vi "PID control - Circle working.vi"() -> ()   [LabVIEW 2017]
uses:
  <vilib>/Simulation/Scripting/Companion Diagram/SimConfigNode/SimParams.ctl
  <vilib>/Simulation/Scripting/Companion Diagram/SimConfigNode/_simSolvers.ctl
  <vilib>/Simulation/Implementation/Shared/SIMSCR Execution Mode.ctl
  <vilib>/Simulation/Param Hierarchy/Typedefs/SIMPH Param Control Actions.ctl
  <vilib>/Simulation/Implementation/Shared/NILVSim_ParamChanged.vi
  <vilib>/Simulation/Implementation/Shared/NILVSIM_BeginStep.vi
  <vilib>/Simulation/Implementation/Shared/NILVSim_Manager.vi
  <vilib>/Utility/error.llb/Clear Errors.vi
  <vilib>/Simulation/Implementation/Shared/NILVSim_FinalizeModel.vi
  <vilib>/DAQmx/read.llb/DAQmx Read (Counter DBL 1Chan 1Samp).vi
  <vilib>/DAQmx/read.llb/DAQmx Read (Digital Bool 1Line 1Point).vi
  917b7e52-755f-4d44-bea8-9e7c9beac24e.vi
  a58f9967-76f1-4ebc-ad3d-26e75a3ca160.vi
  <vilib>/DAQmx/write.llb/DAQmx Write (Analog DBL 1Chan 1Samp).vi
  <vilib>/DAQmx/create/channels.llb/DAQmx Create Channel (AO-Voltage-Basic).vi
  <vilib>/DAQmx/create/channels.llb/DAQmx Create Channel (DI-Digital Input).vi
  <vilib>/DAQmx/create/channels.llb/DAQmx Create Channel (CI-Count Edges).vi
  <vilib>/Simulation/Implementation/Shared/SIM Unbundle Sim Info.vi
  <vilib>/Simulation/Implementation/Shared/NILVSim_Initialize.vi
  <vilib>/Simulation/Utility/Implementation/NILVSim Get Time and IsAcceptedStep.vi
  <vilib>/Simulation/Implementation/Shared/SIMSH Read Queue.vi
  <vilib>/Simulation/Implementation/Shared/NILVSim_GetModelError.vi
  <vilib>/Simulation/Implementation/Shared/SIM Bundle Sim Info.vi
  <vilib>/DAQmx/miscellaneous.llb/DAQmx Fill In Error Info.vi
  <vilib>/Simulation/Implementation/XNodeFramework/SimXNode/SimX.xnode
  <vilib>/Simulation/Model Libraries/PID/SIM PID (Parallel).vi
  <vilib>/Simulation/Model Libraries/PID/SIM PID.vi
  <vilib>/Simulation/Scripting/Companion Diagram/SimConfigNode/SimDog.xnode
  <vilib>/Simulation/Model Libraries/PID/SIM PID (Academic).vi
  <vilib>/Simulation/Implementation/Shared/NI_SIM_Implementation.lvlib
panel:
  out "Boolean":bool
  in  "origin":bool
  out "Previous Y":dbl
  out "Previous X":dbl
  out "Current Y":dbl
  out "Current X":dbl
  out "previous index":dbl
  out "both/reset enter":bool
  out "reset complete":bool
  out "x circle":bool
  out "y circle":bool
  out "Point circle is drawing":dbl=1.0
  out "false":bool
  in  "Radius 2":dbl
  out "No of Points":dbl
  out "Numeric y 2":dbl
  out "Y array":dbl[](array[numeric])
  out "array Y length 2":dbl
  out "Numeric x 2":dbl
  out "X array":dbl[](array[numeric])
  out "array x Length 2":dbl
  in  "stage circle":T1(ring)
  in  "check instruc":bool
  out "x entered":dbl
  out "y enetred":dbl
  out "greater -1 x":bool
  out "less 1 x":bool
  out "direction selected":dbl
  out "at 2f":bool
  out "Step 2J":bool
  out "Step 2H":bool
  out "Shape drawing steps":enum16{"corner", "1st switch", "reverse"}(ring)
  out "Step 2D":bool
  out "Step 2C":bool
  out "c":bool
  in  "height":dbl
  in  "length":dbl
  in  "part":T2(ring)=enum."a"
  out "Step 2A":bool
  out "Step 2B":bool
  in  "Has encoders been reset?":enum16{"don't reset", "reset"}(ring)
  out "x distance currently being travelled":dbl
  out "y distance currently being travelled":dbl
  out "error calced":dbl
  out "p1 dis 2":dbl
  out "p1 dis":dbl
  out "error y":dbl
  out "calc distance y":dbl
  out "calc distanc x":dbl
  out "error x":dbl
  out "reached y":bool
  out "reached x":bool
  out "Numeric":dbl
  in  "Draw rectangle":bool
  in  "Draw circle":bool
  out "In drawing mode":bool
  in  "Right-Down":bool
  in  "Left-Up":bool
  in  "Left-Down":bool
  in  "Right-Up":bool
  in  "right":bool
  in  "left":bool
  in  "motor 2":dbl(slide)=1.5 scale=-10.0..10.0
  in  "down":bool
  in  "up":bool
  in  "Y Length":dbl=30.0
  in  "X Length":dbl=30.0
  in  "Motor 2 encoder":tag="Dev1/ctr1"
  out "Pulses M2":dbl format="%.2f"
  in  "Motor 1 encoder":tag="Dev1/ctr0"
  out "Pulses M1":dbl format="%.2f"
  out "Right":bool
  out "Bottom":bool
  out "Left":bool
  out "Top":bool
  in  "Switch 4/Line 3":tag="Dev1/port0/line3"
  in  "Switch 3/Line 2":tag="Dev1/port0/line2"
  in  "Switch 2/Line 1":tag="Dev1/port0/line1"
  in  "Switch 1/Line 0":tag="Dev1/port0/line0"
  in  "Motor stop":bool
  in  "Motor 1":tag="Dev1/ao0"
  in  "max Voltage":dbl=10.0
  in  "Min Voltage":dbl=-10.0
  in  "Motor 2":tag="Dev1/ao1"
  in  "motor 1":dbl(slide)=1.5 scale=-10.0..10.0
  in  "stop":bool
  # "-1"
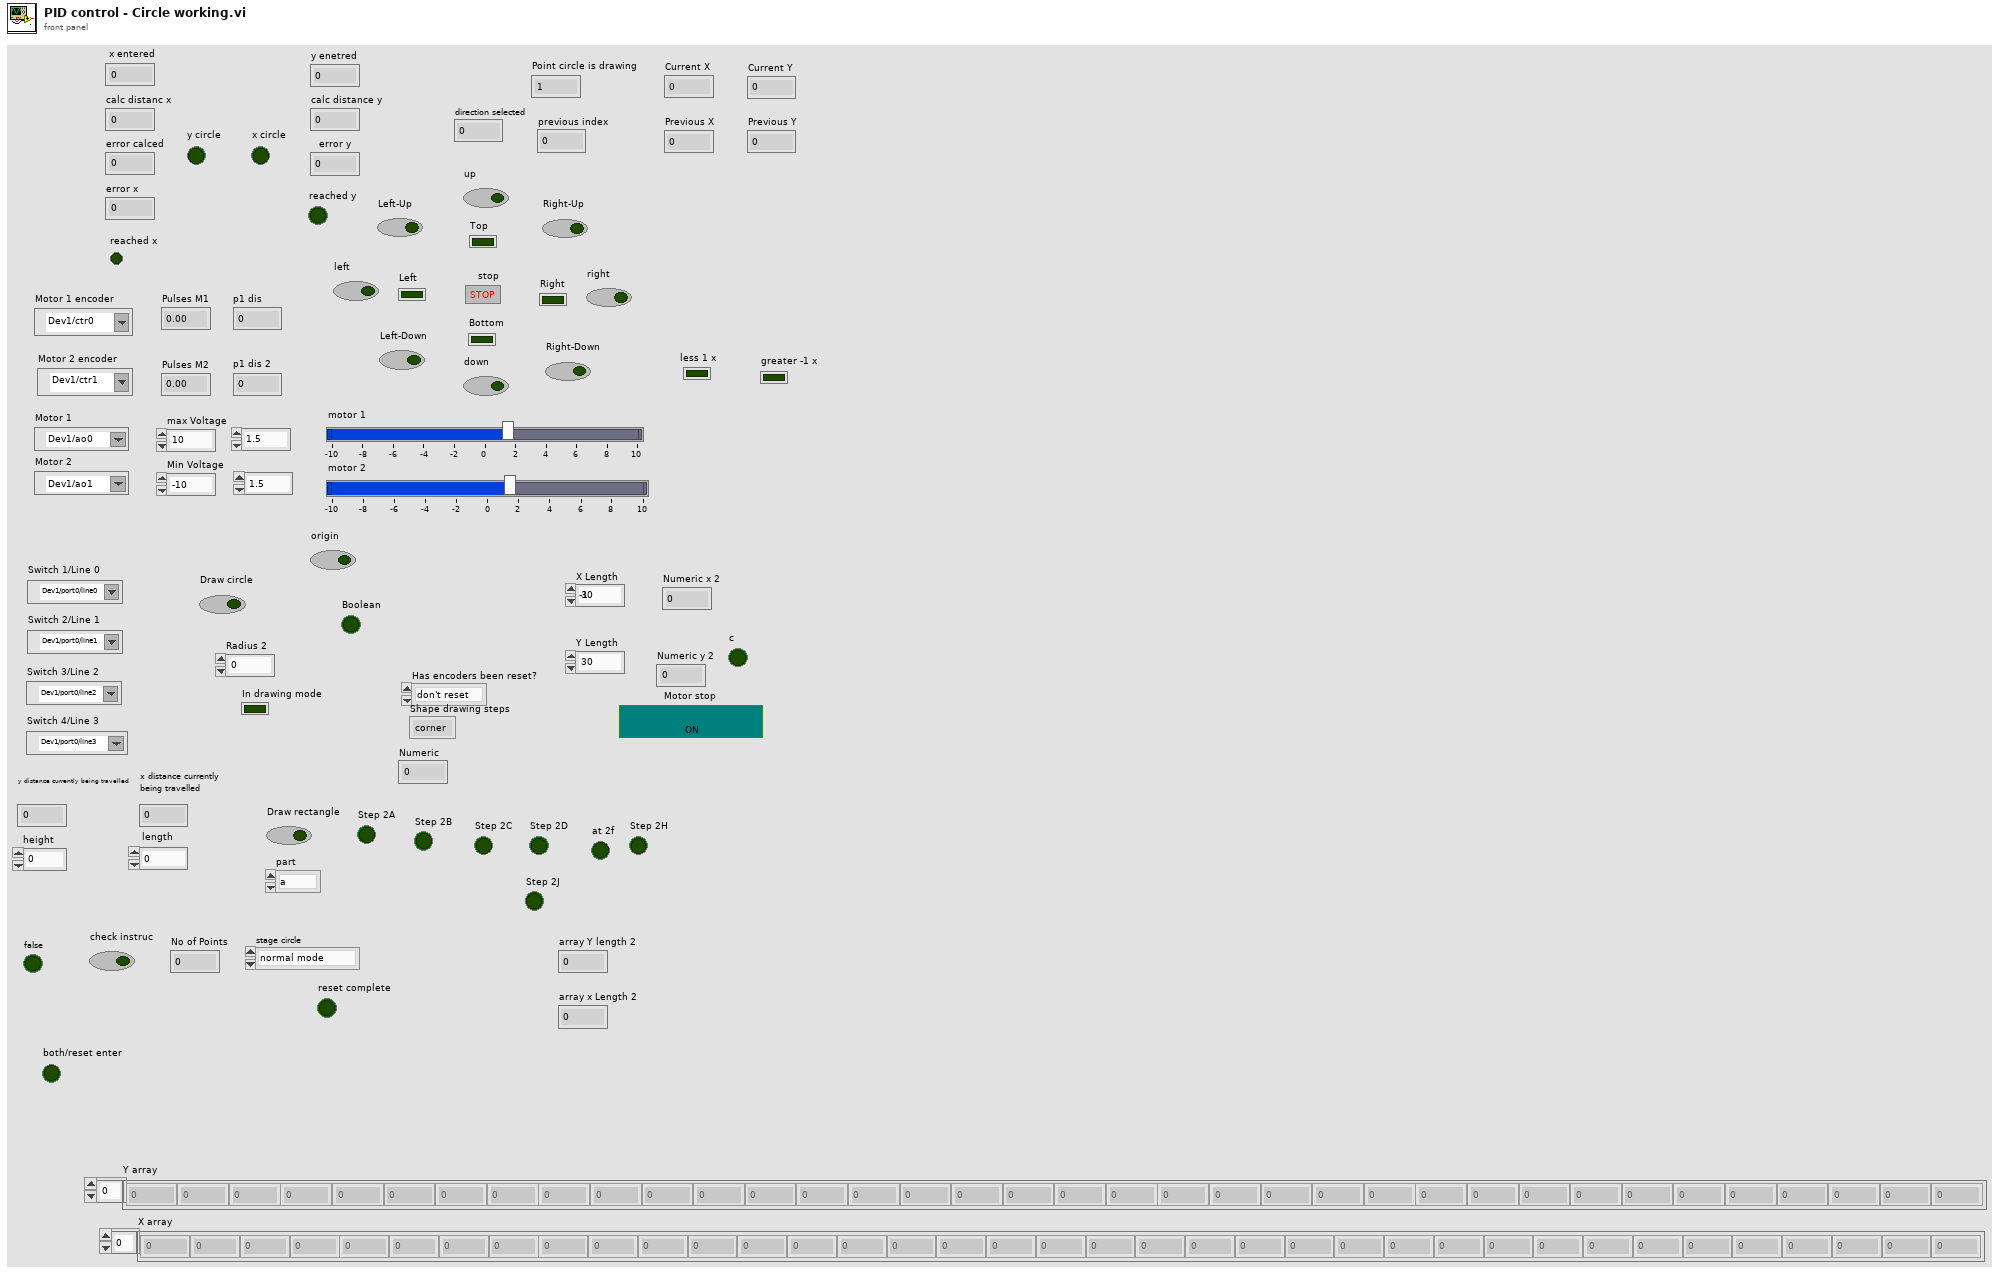
[diagram p1: front panel]
types:
  T1 = enum16{"normal mode", "create points", "draw points", "checking if draw", "reset draw counter"}
  T2 = enum16{"nothing", "j", "i", "h", "g", "f", "e", "d", "c", "b", "a"}
  T3 = enum16{"Simulate to Completion", "Single Time-Step Simulation (Fixed Step Only)"}
  T4 = typedef "SIMSCR Execution Mode.ctl" = enum16{"Simulate to Completion", "Single Time-Step Simulation (Fixed Step Only)"}
  T5 = typedef "SIMPH Param Control Actions.ctl" = enum16{"get params", "set params"}
  T6 = cluster{"SIMSH Sim Time":dbl, "SIM PID Derivative Gain.vi":cluster{"output":dbl}, "SIM PID Derivative Gain.vi - SIMSH":cluster{"SIMSH Sim Time":dbl, "t 3":dbl, "Select 2":cluster{"s? t:f":dbl}, "Equal?":cluster{"x = y?":bool}, "Or":cluster{"x .or. y?":bool}, "Equal To 0?":cluster{"x = 0?":bool}}, "High Frequency [s] (Tf)":dbl, "Gain":cluster{"output":dbl}, "Summation":cluster{"Result":dbl}, "Integral Gain - series.vi":cluster{"output":dbl}, "Integral Gain - series.vi - SIMSH":cluster{"SIMSH Sim Time":dbl, "Select 2":cluster{"s? t:f":dbl}, "integral in gain?":bool, "Integrator":cluster{"output y(t)":dbl}, "Gain 2":cluster{"output":dbl}, "Select":cluster{"s? t:f":dbl}, "Equal To 0?":cluster{"x = 0?":bool}, "Reciprocal":cluster{"1/x":dbl}}}
  T7 = typedef "SimParams.ctl" = cluster{"Initial Time (s)":dbl, "Final Time (s)":dbl, "Step Size (s)":dbl, "ODE Solver":T8, "Minimum Step Size (s)":dbl, "Maximum Step Size (s)":dbl, "Relative Tolerance":dbl, "Absolute Tolerance":dbl, "Software Timing":bool, "Initial Step Size (s)":dbl, "Automatic Fixed Step Size?":bool, "Automatic Discrete Step Size?":bool, "Discrete Step Size (s)":dbl, "Calculate using Time Step":bool, "Solver Wired?":bool, "Prev.Frm.Expected End":u64, "Prev.Frm.Actual End":u64, "Prev.Frm.Finished Late?":bool, "Prev.Iter.Expected End":u64, "Prev.Iter.Actual End":u64, "Prev.Iter.Finished Late?":bool, "Expected Iteration Start":u64, "Actual Iteration Start":u64, "Expected Frame Start":u64, "Actual Frame Start":u64, "Source Name":string, "Name":string, "Period":i64, "Deadline":i64, "Offset":i64, "Start":i64, "Priority":i32, "Timeout":i32, "Processor":i32, "Mode":enum32{"No Change", "Process missed periods, maintain original phase", "Discard missed periods, maintain original phase", "Process missed periods, ignore original phase", "Discard missed periods, ignore original phase"}, "Wakeup reason":enum32{"Normal", "Aborted", "Asynchronous wakeup", "Timing source error", "Timed loop error", "Timeout"}, "Error":errorcluster, "Source Type":string, "Secondary Source Type":string, "Global End Time":u64, "Global Start Time":u64, "Full Solver Reset":bool, "Execution Mode":T4, "Nan/Inf Check":bool, "Custom Solver Library":string, "Solver Is Variable":bool, "custom solver name":string, "Signal Collection Decimation":u32}
  T8 = typedef "_simSolvers.ctl" = enum16{"Runge-Kutta 1 (Euler)", "Runge-Kutta 2", "Runge-Kutta 3", "Runge-Kutta 4", "Runge-Kutta 23 (variable)", "Runge-Kutta 45 (variable)", "BDF (variable)", "Adams-Moulton (variable)", "Rosenbrock (variable)", "Discrete States Only", "SDIRK 4 (variable)", "Radau 5 (variable)", "Radau 9 (variable)", "Radau 13 (variable)", "Radau [Variable Order] (variable)", "Gear's Method (variable)", "Linearizer", "State Query", "Trim Eval", "Custom Solver"}
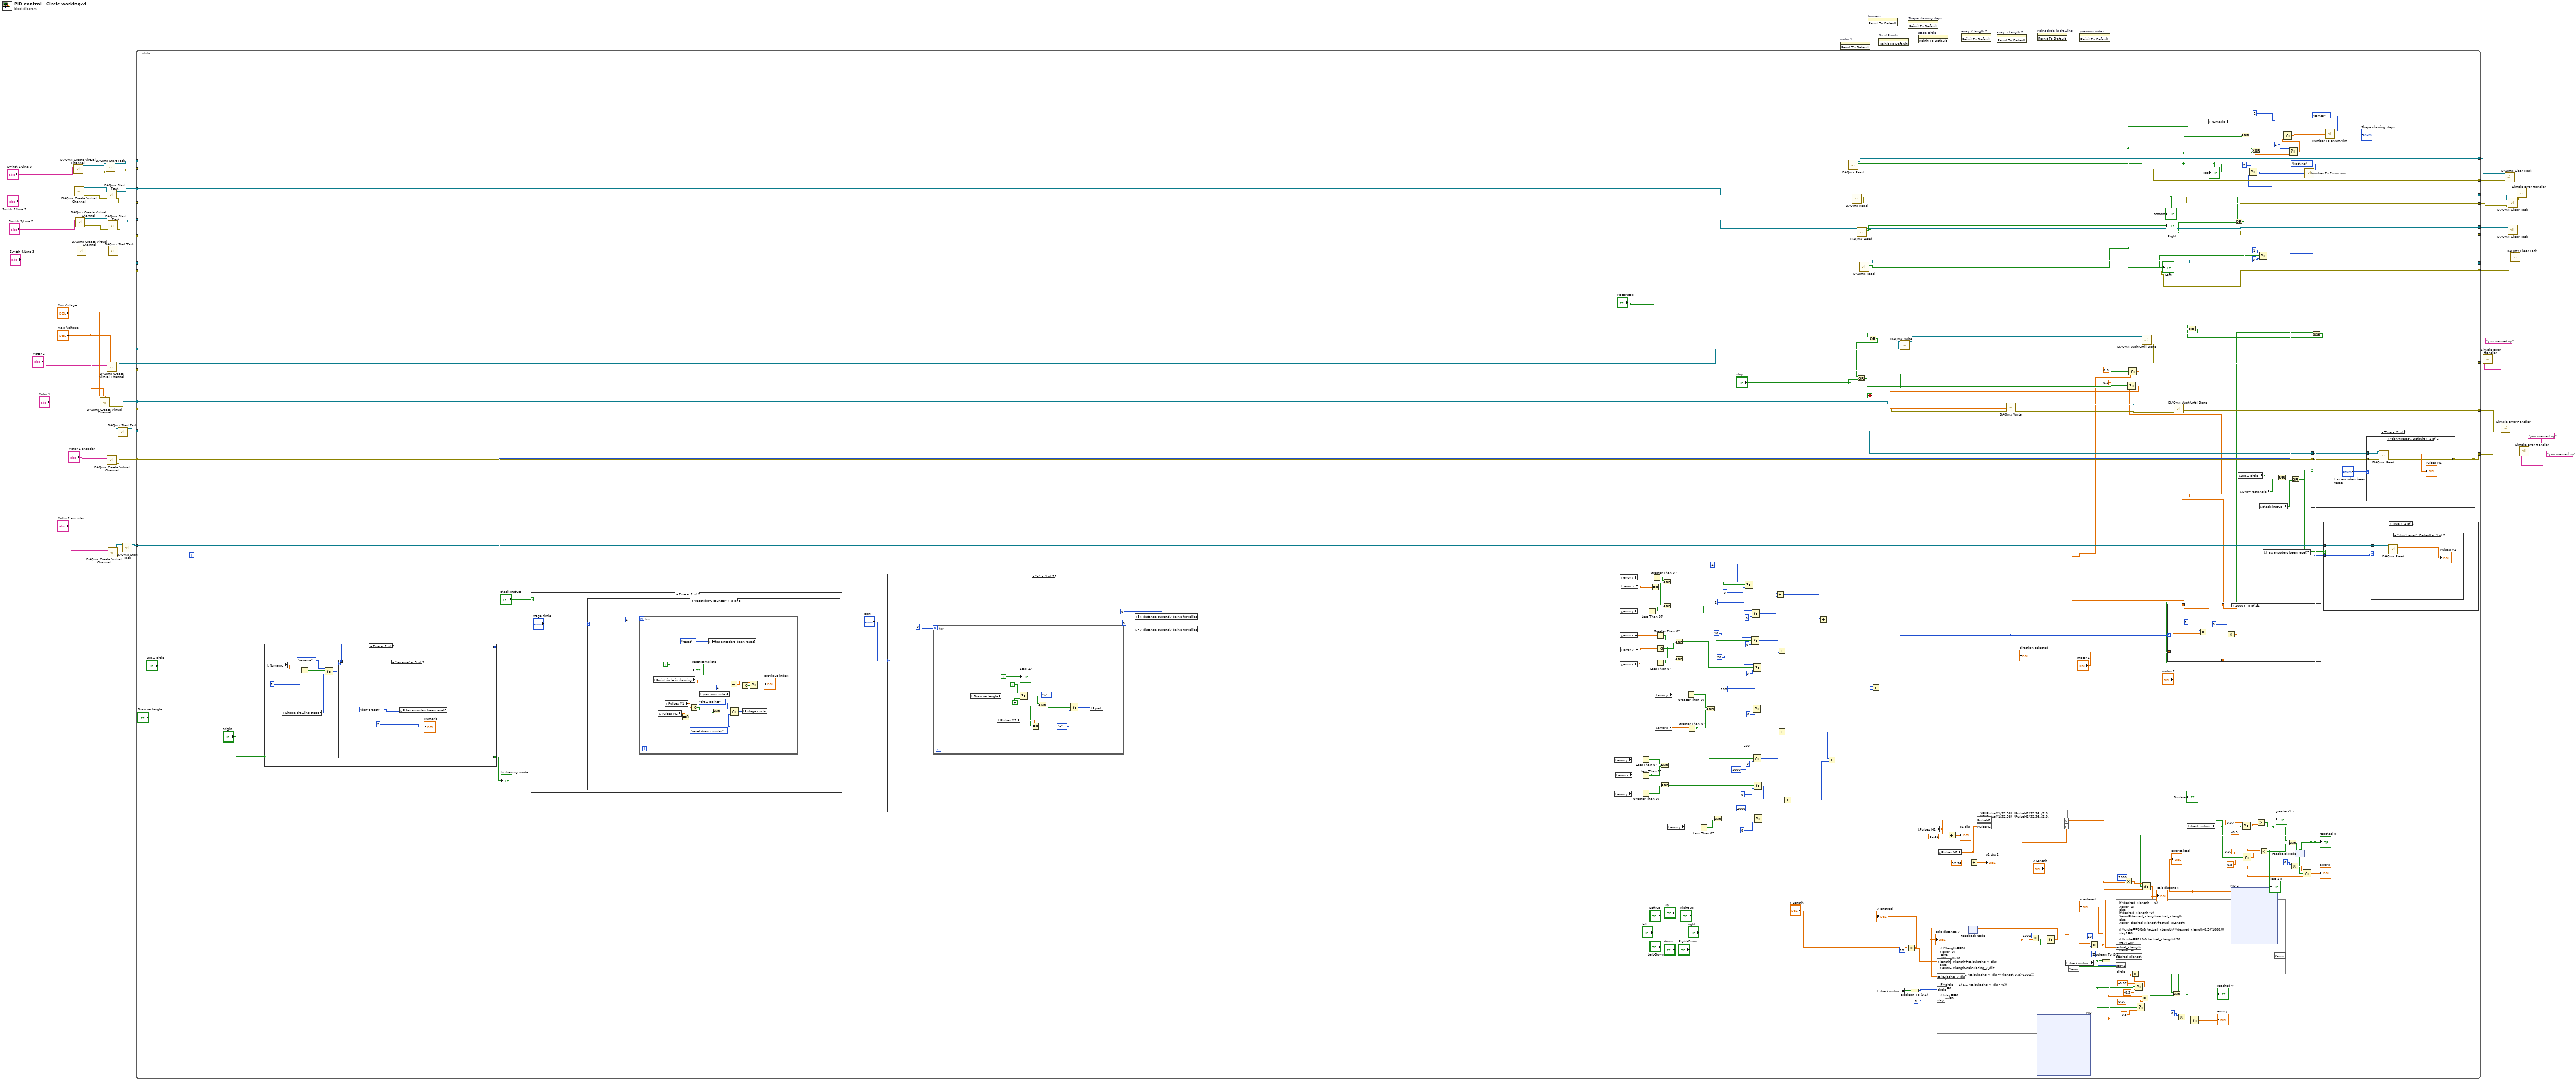
[diagram p0: block diagram]
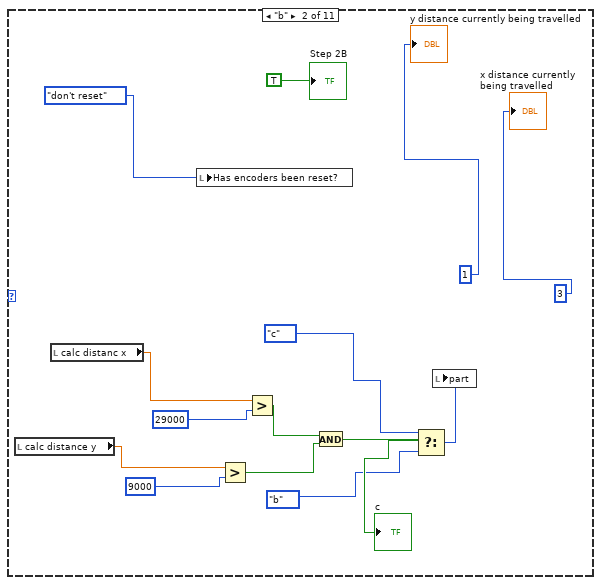
[diagram p2: hidden frame]
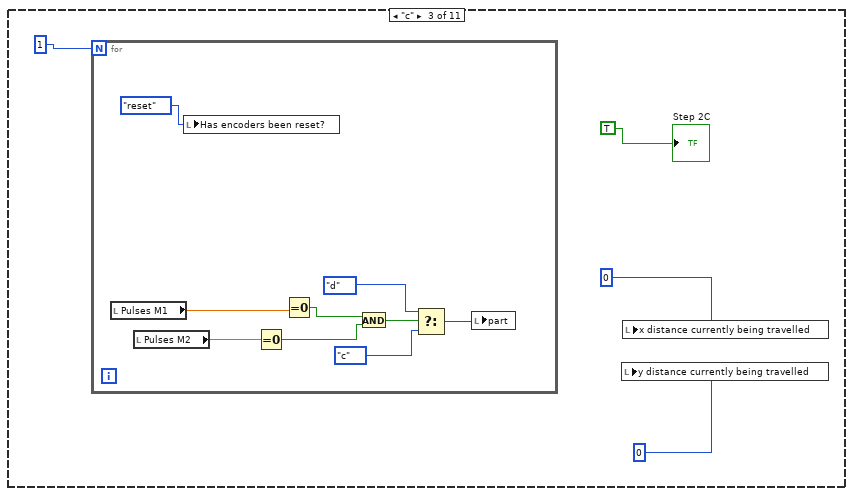
[diagram p3: hidden frame]
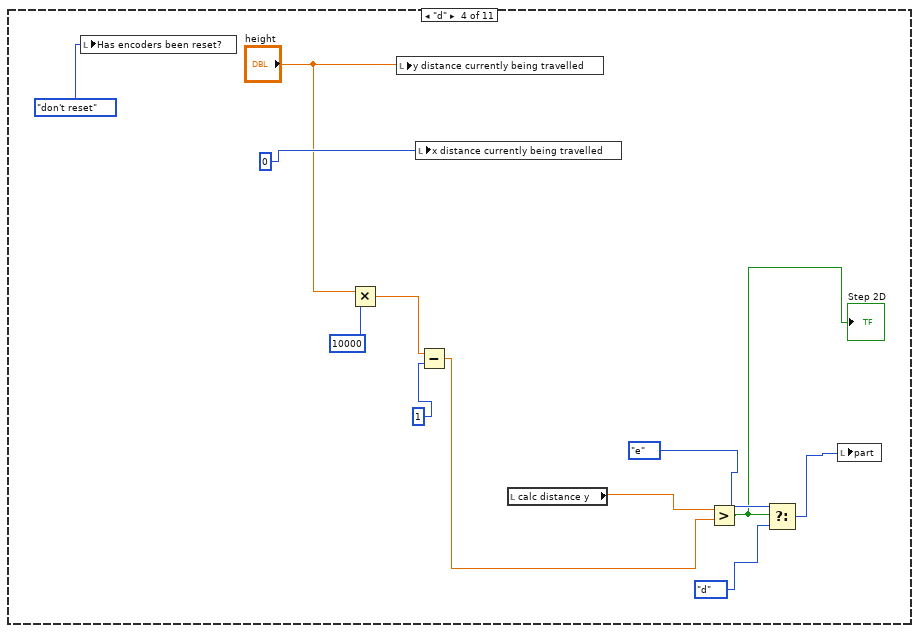
[diagram p4: hidden frame]
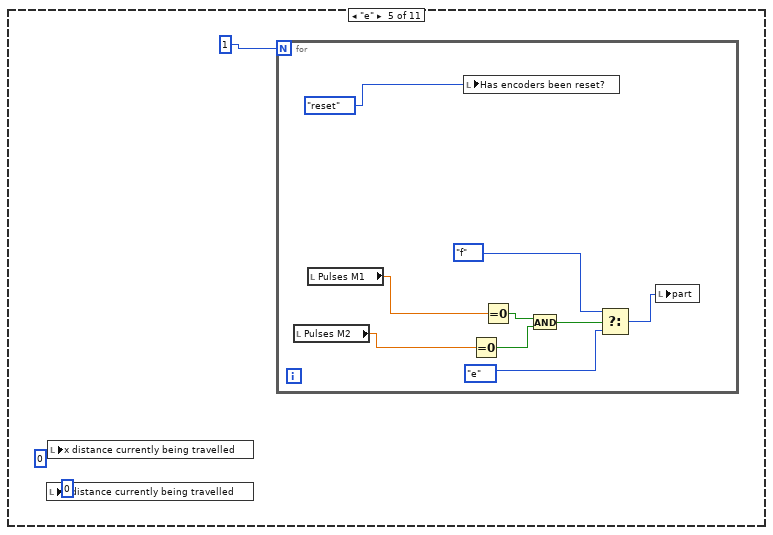
[diagram p5: hidden frame]
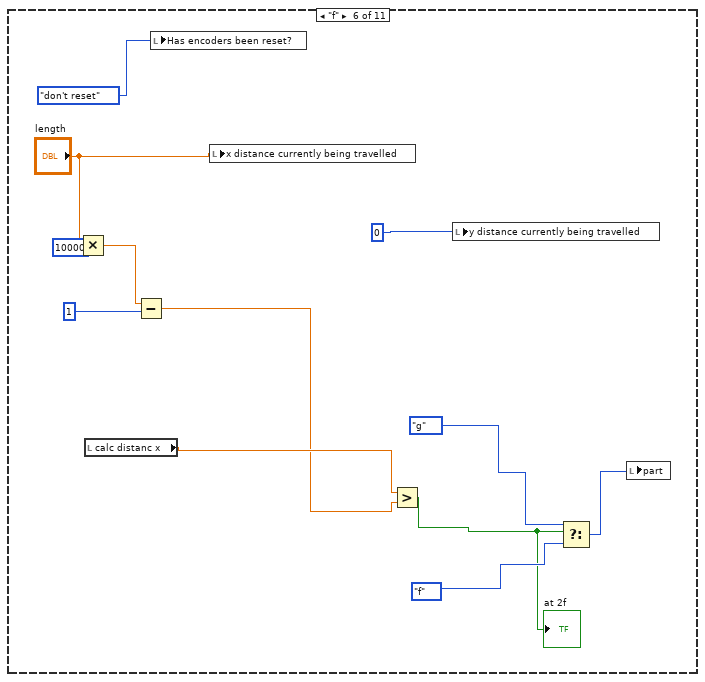
[diagram p6: hidden frame]
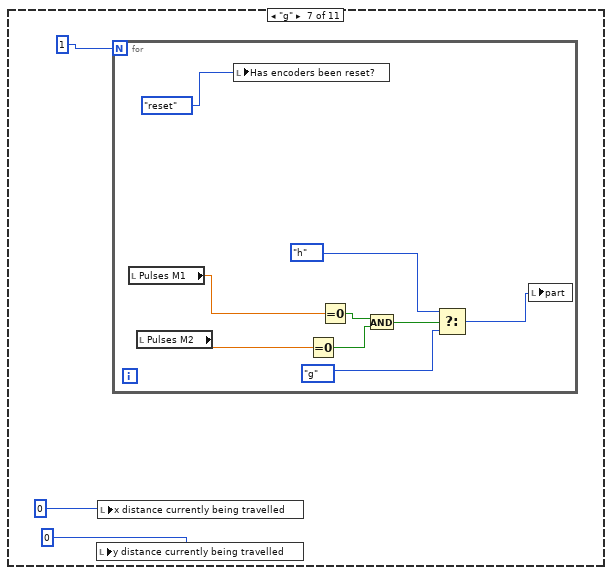
[diagram p7: hidden frame]
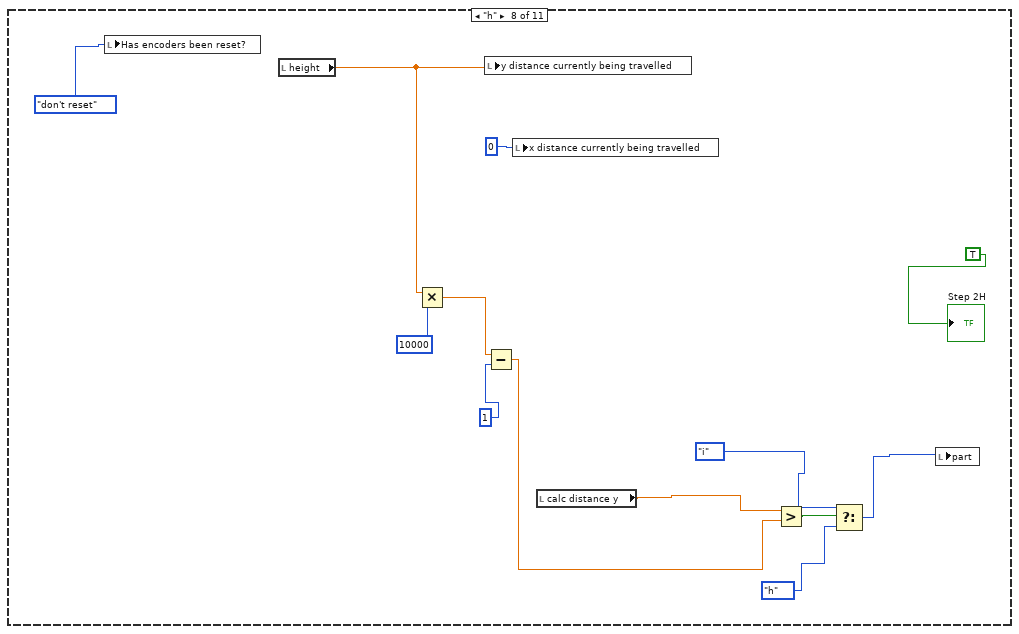
[diagram p8: hidden frame]
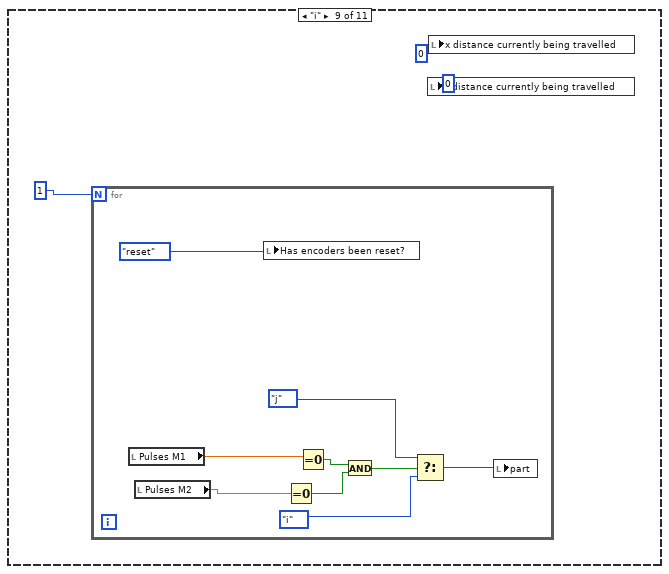
[diagram p9: hidden frame]
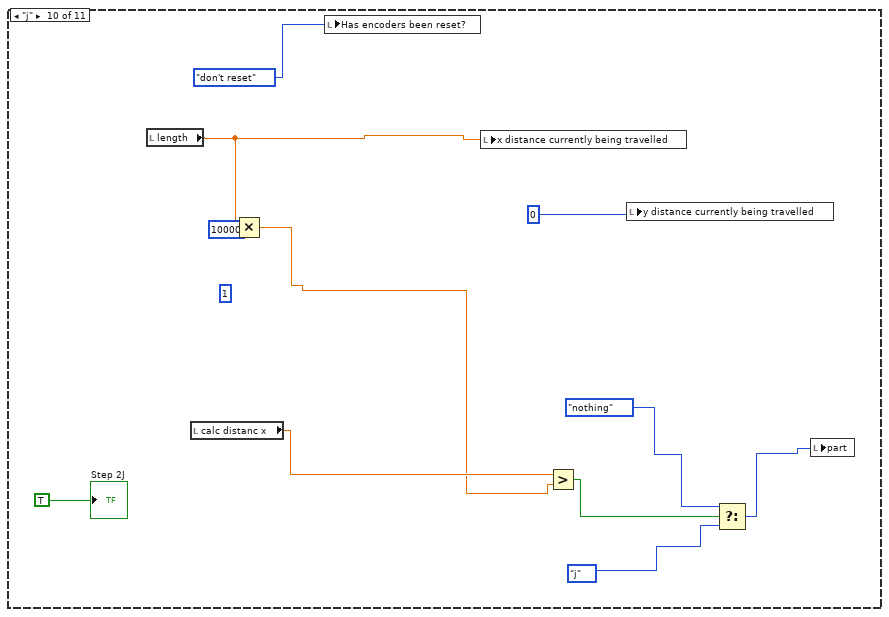
[diagram p10: hidden frame]
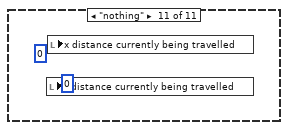
[diagram p11: hidden frame]
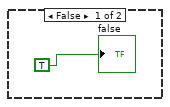
[diagram p12: hidden frame]
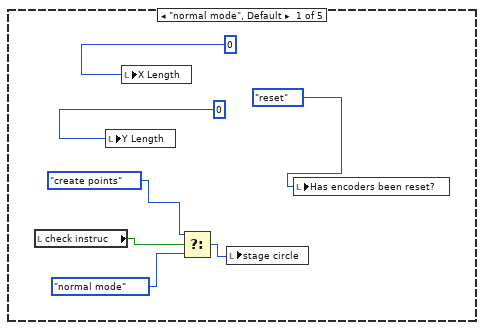
[diagram p13: hidden frame]
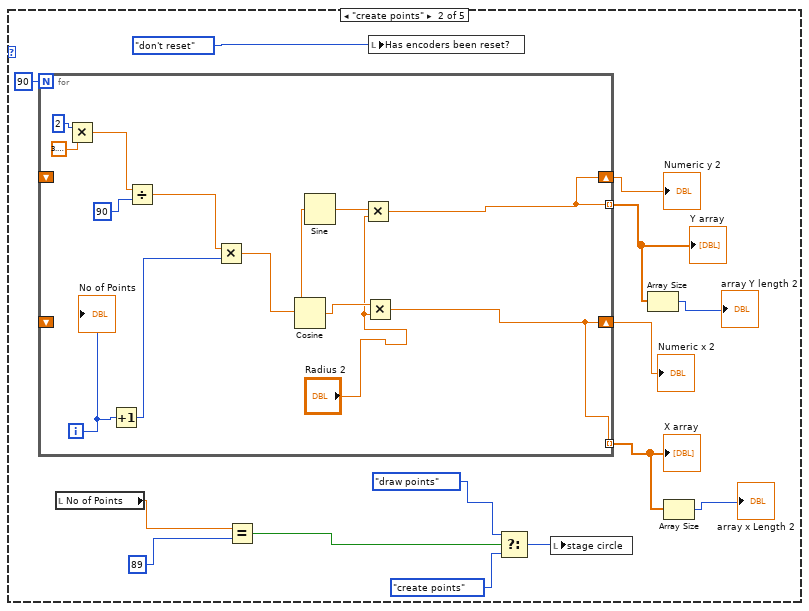
[diagram p14: hidden frame]
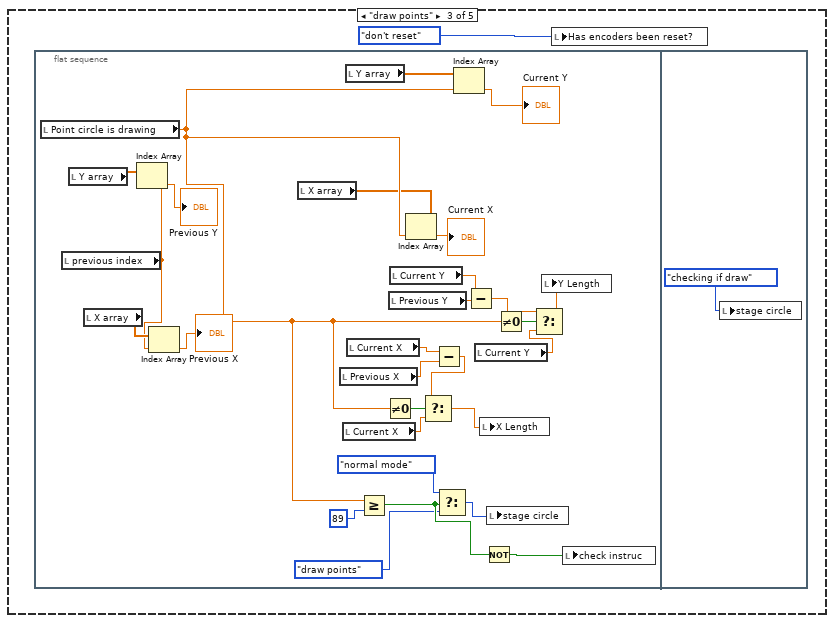
[diagram p15: hidden frame]
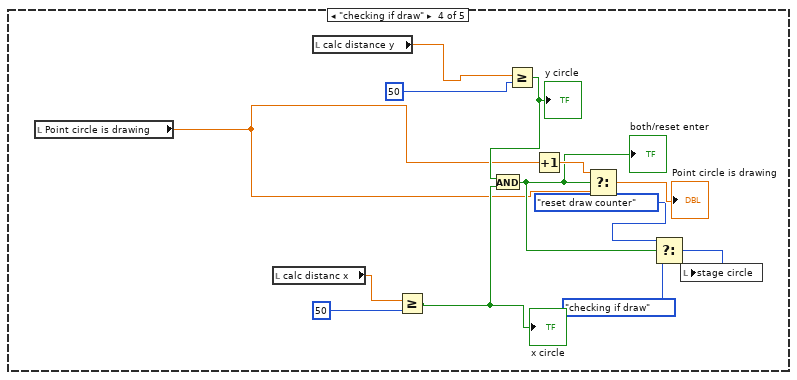
[diagram p16: hidden frame]
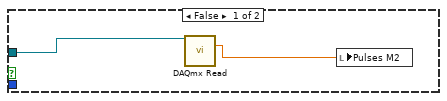
[diagram p17: hidden frame]
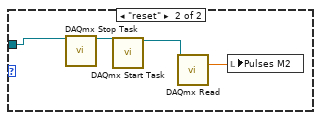
[diagram p18: hidden frame]
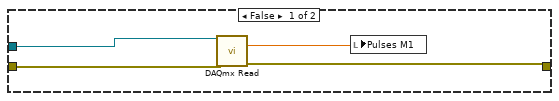
[diagram p19: hidden frame]
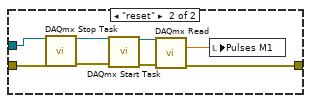
[diagram p20: hidden frame]
diagram:
  n1 = call-poly <vilib>:"DAQmx Create Virtual Channel.vi"("lines"="Switch 1/Line 0") -> ("task out"=w36:refnum<k21>, "error out"=w32:errorcluster)  [unwired: 13 in]
  n2 = call-poly <vilib>:"DAQmx Create Virtual Channel.vi"("lines"="Switch 2/Line 1") -> ("task out"=w35:refnum<k21>, "error out"=w31:errorcluster)  [unwired: 13 in]
  n3 = call-poly <vilib>:"DAQmx Create Virtual Channel.vi"("lines"="Switch 3/Line 2") -> ("task out"=w34:refnum<k21>, "error out"=w30:errorcluster)  [unwired: 13 in]
  n4 = call-poly <vilib>:"DAQmx Create Virtual Channel.vi"("lines"="Switch 4/Line 3") -> ("task out"=w33:refnum<k21>, "error out"=w29:errorcluster)  [unwired: 13 in]
  n5 = call-poly <vilib>:"DAQmx Create Virtual Channel.vi"("maximum value"="max Voltage", "minimum value"="Min Voltage", "physical channels"="Motor 1") -> ("task out"=w46:refnum<k21>, "error out"=w42:errorcluster)  [unwired: 11 in]
  n6 = call <vilib>:"DAQmx Start Task.vi"("task/channels in"=w36, "error in"=w32) -> ("task out"=w28:refnum<k21>, "error out"=w26:errorcluster)  [unwired: 12 in]
  n7 = call <vilib>:"DAQmx Start Task.vi"("task/channels in"=w35, "error in"=w31) -> ("task out"=w24:refnum<k21>, "error out"=w21:errorcluster)  [unwired: 12 in]
  n8 = call-poly <vilib>:"DAQmx Create Virtual Channel.vi"("maximum value"="max Voltage", "minimum value"="Min Voltage", "physical channels"="Motor 2") -> ("task out"=w49:refnum<k21>, "error out"=w41:errorcluster)  [unwired: 11 in]
  n9 = call-poly <vilib>:"DAQmx Create Virtual Channel.vi"("counter"="Motor 1 encoder") -> ("task out"=w7:refnum<k21>, "error out"=w2:errorcluster)  [unwired: 13 in]
  n10 = call-poly <vilib>:"DAQmx Create Virtual Channel.vi"("counter"="Motor 2 encoder") -> ("task out"=w6:refnum<k21>)  [unwired: 13 in, 1 out]
  n11 = call <vilib>:"DAQmx Start Task.vi"("task/channels in"=w34, "error in"=w30) -> ("task out"=w23:refnum<k21>, "error out"=w20:errorcluster)  [unwired: 12 in]
  n12 = call <vilib>:"DAQmx Start Task.vi"("task/channels in"=w33, "error in"=w29) -> ("task out"=w22:refnum<k21>, "error out"=w19:errorcluster)  [unwired: 12 in]
  n13 = call <vilib>:"DAQmx Start Task.vi"("task/channels in"=w7) -> ("task out"=w3:refnum<k21>)  [unwired: 13 in, 1 out]
  n14 = call <vilib>:"DAQmx Start Task.vi"("task/channels in"=w6) -> ("task out"=w1:refnum<k21>)  [unwired: 13 in, 1 out]
  n15 = while {
    tunnel: w49 -> [w245]
    tunnel: [w242] -> w48
    tunnel: w46 -> [w239]
    tunnel: [w238] -> w45
    tunnel: w42 -> [w236]
    tunnel: w41 -> [w235]
    tunnel: w28 -> [w229]
    tunnel: [w228] -> w27
    tunnel: w26 -> [w227]
    tunnel: [w226] -> w25
    tunnel: w24 -> [w225]
    tunnel: w23 -> [w224]
    tunnel: w22 -> [w223]
    tunnel: w21 -> [w222]
    tunnel: w20 -> [w221]
    tunnel: w19 -> [w220]
    tunnel: [w219] -> w18
    tunnel: [w218] -> w17
    tunnel: [w217] -> w16
    tunnel: [w216] -> w15
    tunnel: [w215] -> w14
    tunnel: [w214] -> w13
    tunnel: [w150] -> w10
    tunnel: w3 -> [w152]
    tunnel: w2 -> [w151]
    tunnel: w1 -> [w148]
    stop <- "stop" stop-if-true
    n16 = case shown="True" "check instruc" {
      frame False {
        "false" <- TRUE
      }
      frame True {
        n17 = case shown="\"reset draw counter\"" "stage circle" {
          frame "normal mode", Default {
            n18 = local read "check instruc"() -> (w378:bool)
            n19 = local write "Y Length"(0) -> ()
            n20 = local write "X Length"(0) -> ()
            n21 = Select(t=T1."create points", s=w378, f=T1."normal mode") -> (s? t:f=w379:T1)
            n22 = local write "stage circle"(w379) -> ()
            n23 = local write "Has encoders been reset?"(enum16{"don't reset", "reset"}."reset") -> ()
          }
          frame "create points" {
            n24 = for {
              N: 90 -> [_]
              shift-right: [w398] -> w389
              shift-left: _ -> [_]
              tunnel: [w398] -> w394 mode=indexing
              shift-right: [w397] -> w391
              shift-left: _ -> [_]
              tunnel: [w397] -> w393 mode=indexing
              i -> [w399]
              n25 = Multiply(x=2, y=3.141592653589793) -> (x*y=w402:dbl)
              n26 = Increment(x=w399) -> (x+1=w400:i32)
              n27 = Divide(x=w402, y=90) -> (x/y=w404:dbl)
              n28 = Multiply(x=w404, y=w400) -> (x*y=w401:dbl)
              n29 = Cosine(x=w401) -> (cos(x)=w407:dbl)
              n30 = Sine(x=w401) -> (sin(x)=w408:dbl)
              n31 = Multiply(x=w408, y="Radius 2") -> (x*y=w398:dbl)
              n32 = Multiply(x=w407, y="Radius 2") -> (x*y=w397:dbl)
              "No of Points" <- w399
            }
            "Numeric y 2" <- w389
            "Y array" <- w394
            "Numeric x 2" <- w391
            "X array" <- w393
            n33 = local read "No of Points"() -> (w388:dbl)
            n34 = Equal?(x=w388, y=89) -> (x = y?=w385:bool)
            n35 = local write "Has encoders been reset?"(enum16{"don't reset", "reset"}."don't reset") -> ()
            n36 = Select(t=T1."draw points", s=w385, f=T1."create points") -> (s? t:f=w395:T1)
            n37 = local write "stage circle"(w395) -> ()
            n38 = Array Size(array=w394) -> (size(s)=→"array Y length 2":i32)
            n39 = Array Size(array=w393) -> (size(s)=→"array x Length 2":i32)
          }
          frame "draw points" {
            n40 = flat-sequence {
              frame #0 {
                n41 = local read "Point circle is drawing"() -> (w437:dbl)
                n42 = local read "previous index"() -> (w429:dbl)
                n43 = local read "Y array"() -> (w430:dbl[])
                n44 = local read "X array"() -> (w431:dbl[])
                n45 = Index Array(array=w430, index=w429) -> (element=→"Previous Y":dbl)
                n46 = Index Array(array=w431, index=w429) -> (element=→"Previous X":dbl)
                n47 = local read "X array"() -> (w432:dbl[])
                n48 = local read "Previous X"() -> (w419:dbl)
                n49 = local read "Current X"() -> (w424:dbl)
                n50 = local read "Y array"() -> (w433:dbl[])
                n51 = local read "Current X"() -> (w422:dbl)
                n52 = Greater Or Equal?(x=w437, y=89) -> (x >= y?=w435:bool)
                n53 = Not Equal To 0?(x=w437) -> (x != 0?=w425:bool)
                n54 = local read "Previous Y"() -> (w420:dbl)
                n55 = local read "Current Y"() -> (w421:dbl)
                n56 = Index Array(array=w432, index=w437) -> (element=→"Current X":dbl)
                n57 = Subtract(x=w422, y=w419) -> (x-y=w415:dbl)
                n58 = Select(t=w415, s=w425, f=w424) -> (s? t:f=w412:dbl)
                n59 = Select(t=T1."normal mode", s=w435, f=T1."draw points") -> (s? t:f=w434:T1)
                n60 = Index Array(array=w433, index=w437) -> (element=→"Current Y":dbl)
                n61 = Subtract(x=w421, y=w420) -> (x-y=w414:dbl)
                n62 = local read "Current Y"() -> (w423:dbl)
                n63 = local write "X Length"(w412) -> ()
                n64 = Not(x=w435) -> (.not. x?=w436:bool)
                n65 = local write "stage circle"(w434) -> ()
                n66 = Not Equal To 0?(x=w437) -> (x != 0?=w426:bool)
                n67 = Select(t=w414, s=w426, f=w423) -> (s? t:f=w413:dbl)
                n68 = local write "Y Length"(w413) -> ()
                n69 = local write "check instruc"(w436) -> ()
              }
              frame #1 {
                n70 = local write "stage circle"(T1."checking if draw") -> ()
              }
            }
            n71 = local write "Has encoders been reset?"(enum16{"don't reset", "reset"}."don't reset") -> ()
          }
          frame "checking if draw" {
            n72 = local read "Point circle is drawing"() -> (w439:dbl)
            n73 = local read "calc distanc x"() -> (w447:dbl)
            n74 = local read "calc distance y"() -> (w448:dbl)
            n75 = Greater Or Equal?(x=w447, y=50) -> (x >= y?=w446:bool)
            "x circle" <- w446
            n76 = Greater Or Equal?(x=w448, y=50) -> (x >= y?=w449:bool)
            "y circle" <- w449
            n77 = And(x=w449, y=w446) -> (x .and. y?=w444:bool)
            "both/reset enter" <- w444
            n78 = Increment(x=w439) -> (x+1=w451:dbl)
            n79 = Select(t=w451, s=w444, f=w439) -> (s? t:f=→"Point circle is drawing":dbl)
            n80 = Select(t=T1."reset draw counter", s=w444, f=T1."checking if draw") -> (s? t:f=w445:T1)
            n81 = local write "stage circle"(w445) -> ()
          }
          frame "reset draw counter" {
            n82 = for {
              N: 1 -> [_]
              i -> [w456]
              n83 = local read "Point circle is drawing"() -> (w461:dbl)
              n84 = local read "Pulses M2"() -> (w466:dbl)
              n85 = local read "Pulses M1"() -> (w467:dbl)
              n86 = Equal To 0?(x=w466) -> (x = 0?=w465:bool)
              n87 = Equal To 0?(x=w467) -> (x = 0?=w463:bool)
              n88 = local read "previous index"() -> (w458:dbl)
              n89 = local write "Has encoders been reset?"(enum16{"don't reset", "reset"}."reset") -> ()
              n90 = And(x=w463, y=w465) -> (x .and. y?=w464:bool)
              n91 = Subtract(x=w461, y=1) -> (x-y=w459:dbl)
              n92 = Select(t=T1."draw points", s=w464, f=T1."reset draw counter") -> (s? t:f=w468:T1)
              n93 = Equal To 0?(x=w456) -> (x = 0?=w455:bool)
              n94 = local write "stage circle"(w468) -> ()
              n95 = Select(t=w459, s=w455, f=w458) -> (s? t:f=→"previous index":dbl)
              "reset complete" <- TRUE
            }
          }
        }
      }
    }
    n96 = case shown="\"a\"" "part" {
      frame "a" {
        n97 = for {
          N: 0 -> [_]
          n98 = local read "Draw rectangle"() -> (w249:bool)
          n99 = local read "Pulses M1"() -> (w258:dbl)
          n100 = Select(t=TRUE, s=w249, f=FALSE) -> (s? t:f=w252:bool)
          n101 = Equal To 0?(x=w258) -> (x = 0?=w251:bool)
          n102 = And(x=w252, y=w251) -> (x .and. y?=w250:bool)
          n103 = Select(t=T2."b", s=w250, f=T2."a") -> (s? t:f=w257:T2)
          n104 = local write "part"(w257) -> ()
          "Step 2A" <- TRUE
        }
        n105 = local write "y distance currently being travelled"(0) -> ()
        n106 = local write "x distance currently being travelled"(0) -> ()
      }
      frame "b" {
        n107 = local read "calc distance y"() -> (w260:dbl)
        n108 = local read "calc distanc x"() -> (w261:dbl)
        n109 = local write "Has encoders been reset?"(enum16{"don't reset", "reset"}."don't reset") -> ()
        n110 = Greater?(x=w260, y=9000) -> (0:w266:bool)
        n111 = Greater?(x=w261, y=29000) -> (0:w265:bool)
        n112 = And(x=w265, y=w266) -> (x .and. y?=w264:bool)
        "c" <- w264
        n113 = Select(t=T2."c", s=w264, f=T2."b") -> (s? t:f=w269:T2)
        n114 = local write "part"(w269) -> ()
        "x distance currently being travelled" <- 3
        "y distance currently being travelled" <- 1
        "Step 2B" <- TRUE
      }
      frame "c" {
        n115 = for {
          N: 1 -> [_]
          n116 = local read "Pulses M1"() -> (w285:dbl)
          n117 = local read "Pulses M2"() -> (w281:dbl)
          n118 = local write "Has encoders been reset?"(enum16{"don't reset", "reset"}."reset") -> ()
          n119 = Equal To 0?(x=w281) -> (x = 0?=w279:bool)
          n120 = Equal To 0?(x=w285) -> (x = 0?=w280:bool)
          n121 = And(x=w280, y=w279) -> (x .and. y?=w278:bool)
          n122 = Select(t=T2."d", s=w278, f=T2."c") -> (s? t:f=w284:T2)
          n123 = local write "part"(w284) -> ()
        }
        n124 = local write "y distance currently being travelled"(0) -> ()
        n125 = local write "x distance currently being travelled"(0) -> ()
        "Step 2C" <- TRUE
      }
      frame "d" {
        n126 = local write "Has encoders been reset?"(enum16{"don't reset", "reset"}."don't reset") -> ()
        n127 = Multiply(x="height", y=10000) -> (x*y=w294:dbl)
        n128 = local write "y distance currently being travelled"("height") -> ()
        n129 = local write "x distance currently being travelled"(0) -> ()
        n130 = Subtract(x=w294, y=1) -> (x-y=w291:dbl)
        n131 = local read "calc distance y"() -> (w296:dbl)
        n132 = Greater?(x=w296, y=w291) -> (0:w287:bool)
        "Step 2D" <- w287
        n133 = Select(t=T2."e", s=w287, f=T2."d") -> (s? t:f=w297:T2)
        n134 = local write "part"(w297) -> ()
      }
      frame "e" {
        n135 = local write "y distance currently being travelled"(0) -> ()
        n136 = local write "x distance currently being travelled"(0) -> ()
        n137 = for {
          N: 1 -> [_]
          n138 = local read "Pulses M2"() -> (w303:dbl)
          n139 = local read "Pulses M1"() -> (w304:dbl)
          n140 = local write "Has encoders been reset?"(enum16{"don't reset", "reset"}."reset") -> ()
          n141 = Equal To 0?(x=w303) -> (x = 0?=w309:bool)
          n142 = Equal To 0?(x=w304) -> (x = 0?=w310:bool)
          n143 = And(x=w310, y=w309) -> (x .and. y?=w308:bool)
          n144 = Select(t=T2."f", s=w308, f=T2."e") -> (s? t:f=w302:T2)
          n145 = local write "part"(w302) -> ()
        }
      }
      frame "f" {
        n146 = Multiply(x="length", y=10000) -> (x*y=w317:dbl)
        n147 = local read "calc distanc x"() -> (w320:dbl)
        n148 = Subtract(x=w317, y=1) -> (x-y=w314:dbl)
        n149 = local write "Has encoders been reset?"(enum16{"don't reset", "reset"}."don't reset") -> ()
        n150 = local write "x distance currently being travelled"("length") -> ()
        n151 = Greater?(x=w320, y=w314) -> (0:w311:bool)
        "at 2f" <- w311
        n152 = local write "y distance currently being travelled"(0) -> ()
        n153 = Select(t=T2."g", s=w311, f=T2."f") -> (s? t:f=w319:T2)
        n154 = local write "part"(w319) -> ()
      }
      frame "g" {
        n155 = local write "y distance currently being travelled"(0) -> ()
        n156 = local write "x distance currently being travelled"(0) -> ()
        n157 = for {
          N: 1 -> [_]
          n158 = local read "Pulses M1"() -> (w327:dbl)
          n159 = local read "Pulses M2"() -> (w326:dbl)
          n160 = local write "Has encoders been reset?"(enum16{"don't reset", "reset"}."reset") -> ()
          n161 = Equal To 0?(x=w326) -> (x = 0?=w333:bool)
          n162 = Equal To 0?(x=w327) -> (x = 0?=w334:bool)
          n163 = And(x=w334, y=w333) -> (x .and. y?=w332:bool)
          n164 = Select(t=T2."h", s=w332, f=T2."g") -> (s? t:f=w329:T2)
          n165 = local write "part"(w329) -> ()
        }
      }
      frame "h" {
        n166 = local write "Has encoders been reset?"(enum16{"don't reset", "reset"}."don't reset") -> ()
        n167 = local read "height"() -> (w338:dbl)
        n168 = Multiply(x=w338, y=10000) -> (x*y=w346:dbl)
        n169 = local write "y distance currently being travelled"(w338) -> ()
        n170 = Subtract(x=w346, y=1) -> (x-y=w343:dbl)
        n171 = local write "x distance currently being travelled"(0) -> ()
        n172 = local read "calc distance y"() -> (w336:dbl)
        n173 = Greater?(x=w336, y=w343) -> (0:w347:bool)
        n174 = Select(t=T2."i", s=w347, f=T2."h") -> (s? t:f=w339:T2)
        n175 = local write "part"(w339) -> ()
        "Step 2H" <- TRUE
      }
      frame "i" {
        n176 = for {
          N: 1 -> [_]
          n177 = local read "Pulses M1"() -> (w353:dbl)
          n178 = local read "Pulses M2"() -> (w352:dbl)
          n179 = local write "Has encoders been reset?"(enum16{"don't reset", "reset"}."reset") -> ()
          n180 = Equal To 0?(x=w352) -> (x = 0?=w358:bool)
          n181 = Equal To 0?(x=w353) -> (x = 0?=w359:bool)
          n182 = And(x=w359, y=w358) -> (x .and. y?=w357:bool)
          n183 = Select(t=T2."j", s=w357, f=T2."i") -> (s? t:f=w351:T2)
          n184 = local write "part"(w351) -> ()
        }
        n185 = local write "y distance currently being travelled"(0) -> ()
        n186 = local write "x distance currently being travelled"(0) -> ()
      }
      frame "j" {
        (unwired) 1
        n187 = local read "length"() -> (w363:dbl)
        n188 = local read "calc distanc x"() -> (w365:dbl)
        n189 = Multiply(x=w363, y=10000) -> (x*y=w360:dbl)
        n190 = local write "Has encoders been reset?"(enum16{"don't reset", "reset"}."don't reset") -> ()
        n191 = local write "x distance currently being travelled"(w363) -> ()
        n192 = Greater?(x=w365, y=w360) -> (0:w368:bool)
        n193 = local write "y distance currently being travelled"(0) -> ()
        n194 = Select(t=T2."nothing", s=w368, f=T2."j") -> (s? t:f=w364:T2)
        n195 = local write "part"(w364) -> ()
        "Step 2J" <- TRUE
      }
      frame "nothing" {
        n196 = local write "y distance currently being travelled"(0) -> ()
        n197 = local write "x distance currently being travelled"(0) -> ()
      }
    }
    n198 = local read "error y"() -> (w122:dbl)
    n199 = local read "error y"() -> (w121:dbl)
    n200 = local read "error x"() -> (w123:dbl)
    n201 = local read "error y"() -> (w137:dbl)
    n202 = local read "error y"() -> (w134:dbl)
    n203 = local read "error x"() -> (w130:dbl)
    n204 = local read "error x"() -> (w129:dbl)
    n205 = local read "error y"() -> (w138:dbl)
    n206 = local read "error x"() -> (w139:dbl)
    n207 = Less Than 0?(x=w122) -> (x < 0?=w120:bool)
    n208 = Less Than 0?(x=w123) -> (x < 0?=w119:bool)
    n209 = Greater Than 0?(x=w121) -> (x > 0?=w118:bool)
    n210 = Less Than 0?(x=w134) -> (x < 0?=w132:bool)
    n211 = Equal To 0?(x=w139) -> (x = 0?=w133:bool)
    n212 = Greater Than 0?(x=w137) -> (x > 0?=w136:bool)
    n213 = local read "error y"() -> (w115:dbl)
    n214 = local read "error x"() -> (w114:dbl)
    n215 = Greater Than 0?(x=w130) -> (x > 0?=w128:bool)
    n216 = Equal To 0?(x=w138) -> (x = 0?=w127:bool)
    n217 = Less Than 0?(x=w129) -> (x < 0?=w126:bool)
    n218 = And(x=w120, y=w119) -> (x .and. y?=w116:bool)
    n219 = And(x=w119, y=w118) -> (x .and. y?=w117:bool)
    n220 = And(x=w136, y=w133) -> (x .and. y?=w135:bool)
    n221 = And(x=w133, y=w132) -> (x .and. y?=w131:bool)
    n222 = local read "error y"() -> (w110:dbl)
    n223 = And(x=w128, y=w127) -> (x .and. y?=w125:bool)
    n224 = And(x=w127, y=w126) -> (x .and. y?=w124:bool)
    n225 = Greater Than 0?(x=w115) -> (x > 0?=w113:bool)
    n226 = Greater Than 0?(x=w114) -> (x > 0?=w111:bool)
    n227 = Less Than 0?(x=w110) -> (x < 0?=w109:bool)
    n228 = And(x=w113, y=w111) -> (x .and. y?=w112:bool)
    n229 = And(x=w111, y=w109) -> (x .and. y?=w108:bool)
    n230 = Select(t=1, s=w135, f=0) -> (s? t:f=w198:i32)
    n231 = Select(t=10, s=w124, f=0) -> (s? t:f=w196:i32)
    n232 = Select(t=2, s=w131, f=0) -> (s? t:f=w197:i32)
    n233 = Select(t=100, s=w112, f=0) -> (s? t:f=w194:i32)
    n234 = Select(t=200, s=w116, f=0) -> (s? t:f=w193:i32)
    n235 = Select(t=20, s=w125, f=0) -> (s? t:f=w195:i32)
    n236 = Select(t=1000, s=w117, f=0) -> (s? t:f=w192:i32)
    n237 = Select(t=2000, s=w108, f=0) -> (s? t:f=w178:i32)
    n238 = Add(x=w198, y=w197) -> (x+y=w191:i32)
    n239 = Add(x=w196, y=w195) -> (x+y=w190:i32)
    n240 = Add(x=w194, y=w193) -> (x+y=w189:i32)
    n241 = Add(x=w192, y=w178) -> (x+y=w177:i32)
    n242 = Add(x=w191, y=w190) -> (x+y=w188:i32)
    n243 = Add(x=w189, y=w177) -> (x+y=w176:i32)
    n244 = call-poly <vilib>:"DAQmx Read.vi"("task/channels in"=w229, "error in"=w227) -> ("task out"=w228:refnum<k21>, "data"=w160:bool, "error out"=w226:errorcluster)  [unwired: 11 in]
    "Top" <- w160
    n245 = call-poly <vilib>:"DAQmx Read.vi"("task/channels in"=w225, "error in"=w222) -> ("task out"=w219:refnum<k21>, "data"=w169:bool, "error out"=w216:errorcluster)  [unwired: 11 in]
    "Bottom" <- w169
    n246 = call-poly <vilib>:"DAQmx Read.vi"("task/channels in"=w224, "error in"=w221) -> ("task out"=w218:refnum<k21>, "data"=w168:bool, "error out"=w215:errorcluster)  [unwired: 11 in]
    "Right" <- w168
    n247 = call-poly <vilib>:"DAQmx Read.vi"("task/channels in"=w223, "error in"=w220) -> ("task out"=w217:refnum<k21>, "data"=w167:bool, "error out"=w214:errorcluster)  [unwired: 11 in]
    "Left" <- w167
    n248 = Add(x=w188, y=w176) -> (x+y=w107:i32)
    "direction selected" <- w107
    n249 = local read "check instruc"() -> (w67:bool)
    n250 = Multiply(x="Y Length", y=10) -> (x*y=w83:dbl)
    "y enetred" <- w83
    n251 = Boolean To (0,1)(Boolean=w67) -> (0, 1=w66:i16)
    n252 = local read "Pulses M1"() -> (w149:dbl)
    n253 = local read "Pulses M2"() -> (w153:dbl)
    n254 = Divide(x=w149, y=52.56) -> (x/y=→"p1 dis":dbl)
    n255 = feedback #1() -> (w76:dbl)  [unwired: 1 in]
    "calc distance y" <- w76
    n256 = formula code="if (Ylength==0)\nYerror=0;\n else  \nif(Ylength<0)\nYerror= Ylength+calculating_y_dis;\nelse\nYerror= Ylength-calculating_y_dis;\n\nif ((circle==0)&& (calculating_y_dis>((Ylength-0.5)*1000)))\nstay=0;\n\nif ((circle==1) && (calculating_y_dis>70))\nstay=0;\n\nif (stay==0 )\nYerror=0;"("Ylength"=w83, "calculating_y_dis"=w76, "stay"=1, "circle"=w66) -> ("Yerror"=w141:dbl)
    n257 = Divide(x=w153, y=52.56) -> (x/y=→"p1 dis 2":dbl)
    n258 = formula code="X=((PulseM1/52.56)+(PulseM2/52.56))/2.0;\nY=((PulseM1/52.56)+(PulseM2/52.56))/2.0;"("PulseM1"=w149, "PulseM2"=w153) -> ("X"=w80:dbl, "Y"=w81:dbl)
    n259 = Multiply(x=1000, y=w81) -> (x*y=w97:dbl)
    n260 = xnode "PID"("Error"=w141) -> ("Output"=w71:dbl)  [unwired: 2 in, 11 out]
    n261 = local read "check instruc"() -> (w62:bool)
    n262 = Multiply(x="X Length", y=10) -> (x*y=w86:dbl)
    "x entered" <- w86
    n263 = Boolean To (0,1)(Boolean=w62) -> (0, 1=w65:i16)
    n264 = Multiply(x=1000, y=w80) -> (x*y=w93:dbl)
    n265 = Select(t=-0.07, s=w62, f=-0.5) -> (s? t:f=w61:dbl)
    n266 = Greater?(x=w71, y=w61) -> (0:w106:bool)
    n267 = Select(t=0.07, s=w62, f=0.5) -> (s? t:f=w60:dbl)
    n268 = Less?(x=w71, y=w60) -> (x < y?=w105:bool)
    n269 = case shown="2000" w107 {
      tunnel: "motor 1" -> [w1021 w1024 w1027 w1034 w1038 w1042 w1048 w1054 w1060 w1065 w1072]
      tunnel: "motor 2" -> [w1018 w1026 w1029 w1032 w1037 w1040 w1046 w1052 w1058 w1066 w1071]
      tunnel: [w1017 w1026 w1028 w1031 w1037 w1039 w1045 w1051 w1057 w1063 w1070] -> w84
      tunnel: [w1020 w1023 w1027 w1033 w1038 w1041 w1047 w1053 w1059 w1064 w1069] -> w85
      frame 0, Default {
        n270 = Multiply(x=0, y=w1021) -> (x*y=w1020:dbl)
        n271 = Multiply(x=0, y=w1018) -> (x*y=w1017:dbl)
      }
      frame 1 {
        n272 = Multiply(x=-1, y=w1024) -> (x*y=w1023:dbl)
      }
      frame 2 {
        n273 = Multiply(x=-1.003, y=w1029) -> (x*y=w1028:dbl)
      }
      frame 10 {
        n274 = Multiply(x=-1, y=w1034) -> (x*y=w1033:dbl)
        n275 = Multiply(x=-1.1, y=w1032) -> (x*y=w1031:dbl)
      }
      frame 20 {
      }
      frame 100 {
        n276 = Multiply(x=0, y=w1042) -> (x*y=w1041:dbl)
        n277 = Multiply(x=1, y=w1040) -> (x*y=w1039:dbl)
      }
      frame 200 {
        n278 = Multiply(x=0, y=w1048) -> (x*y=w1047:dbl)
        n279 = Multiply(x=-1, y=w1046) -> (x*y=w1045:dbl)
      }
      frame 1000 {
        n280 = Multiply(x=-1, y=w1054) -> (x*y=w1053:dbl)
        n281 = Multiply(x=0, y=w1052) -> (x*y=w1051:dbl)
      }
      frame 2000 {
        n282 = Multiply(x=1, y=w1060) -> (x*y=w1059:dbl)
        n283 = Multiply(x=0, y=w1058) -> (x*y=w1057:dbl)
      }
      frame 4000 {
        n284 = Multiply(x=-1, y=w1065) -> (x*y=w1064:dbl)
        n285 = Multiply(x=0, y=w1066) -> (x*y=w1063:dbl)
      }
      frame 8000 {
        n286 = Multiply(x=-1, y=w1072) -> (x*y=w1069:dbl)
        n287 = Multiply(x=0, y=w1071) -> (x*y=w1070:dbl)
      }
    }
    n288 = And(x=w106, y=w105) -> (x .and. y?=w96:bool)
    "reached y" <- w96
    n289 = Select(t=w97, s=w96, f=w81) -> (s? t:f=w95:dbl)
    n290 = feedback-in #1(w95) -> ()
    n291 = Multiply(x=0, y=w71) -> (x*y=w104:dbl)
    n292 = local read "check instruc"() -> (w51:bool)
    "Boolean" <- w51
    n293 = Select(t=w104, s=w96, f=w71) -> (s? t:f=→"error y":dbl)
    n294 = local read "Numeric"() -> (w143:dbl)
    n295 = Or(x=w169, y=w168) -> (x .or. y?=w212:bool)
    n296 = local read "Draw circle"() -> (w147:bool)
    n297 = local read "Draw rectangle"() -> (w146:bool)
    n298 = And(x=w167, y=w160) -> (x .and. y?=w144:bool)
    n299 = Select(t=-0.07, s=w51, f=-0.5) -> (s? t:f=w55:dbl)
    n300 = Select(t=0.07, s=w51, f=0.5) -> (s? t:f=w52:dbl)
    n301 = Exclusive Or(1:w160, 2:w167) -> (0:w174:bool)
    n302 = Select(t=1, s=w167, f=0) -> (s? t:f=w159:i32)
    n303 = Select(t=2, s=w160, f=w159) -> (s? t:f=w164:i32)
    n304 = local read "check instruc"() -> (w74:bool)
    n305 = local read "Has encoders been reset?"() -> (w79:enum16{"don't reset", "reset"})
    n306 = Or(x=w147, y=w146) -> (x .or. y?=w73:bool)
    n307 = Select(t=1, s=w174, f=w143) -> (s? t:f=w173:dbl)
    n308 = Select(t=2, s=w144, f=w173) -> (s? t:f=w171:dbl)
    n309 = Or(x=w73, y=w74) -> (x .or. y?=w72:bool)
    n310 = feedback #2() -> (w91:bool)  [unwired: 1 in]
    "reached x" <- w91
    n311 = Select(t=w93, s=w91, f=w80) -> (s? t:f=w75:dbl)
    "calc distanc x" <- w75
    n312 = formula code="if (desired_xlength==0)\nXerror=0;\nelse\nif(desired_xlength>0)\nXerror=desired_xlength-actual_xLength;\nelse\nXerror=desired_xlength+actual_xLength;\n\nif ((circle==0)&& (actual_xLength>((desired_xlength-0.5)*1000)))\nstay1=0;\n\nif ((circle==1) && (actual_xLength>70))\nstay1=0;\nif (stay1==0)\nXerror=0;"("actual_xLength"=w75, "desired_xlength"=w86, "stay1"=1, "circle"=w65) -> ("Xerror"=w140:dbl)
    "error calced" <- w140
    n313 = xnode "PID 2"("Error"=w140) -> ("Output"=w70:dbl)  [unwired: 2 in, 11 out]
    n314 = Greater?(x=w70, y=w55) -> (0:w89:bool)
    "greater -1 x" <- w89
    n315 = Less?(x=w70, y=w52) -> (x < y?=w90:bool)
    "less 1 x" <- w90
    n316 = And(x=w89, y=w90) -> (x .and. y?=w92:bool)
    n317 = Multiply(x=0, y=w70) -> (x*y=w101:dbl)
    n318 = feedback-in #2(w92) -> ()
    n319 = Select(t=w101, s=w91, f=w70) -> (s? t:f=→"error x":dbl)
    n320 = call "Number To Enum.vim"("number"=w164, "enum type"=enum16{"Nothing", "Left", "Top"}."Nothing") -> ("number as enum"=w161:enum16{"Nothing", "Left", "Top"})
    n321 = case shown="True" "origin" {
      selector: "origin" -> [w994 w1002]
      tunnel: [w994 w1002] -> w175
      tunnel: w161 -> [_ w995]
      frame False {
      }
      frame True {
        n322 = local read "Numeric"() -> (w1000:dbl)
        n323 = local read "Shape drawing steps"() -> (w997:enum16{"corner", "1st switch", "reverse"})
        n324 = Equal?(x=w1000, y=2) -> (x = y?=w999:bool)
        n325 = Select(t=enum16{"corner", "1st switch", "reverse"}."reverse", s=w999, f=w997) -> (s? t:f=w996:enum16{"corner", "1st switch", "reverse"})
        n326 = case shown="\"reverse\"" w996 {
          tunnel: w995 -> [_ w1006 _]
          frame "corner" {
            n327 = local write "Y Length"(50) -> ()
            n328 = local write "Has encoders been reset?"(enum16{"don't reset", "reset"}."don't reset") -> ()
            n329 = local write "X Length"(-50) -> ()
          }
          frame "1st switch" {
            n330 = case shown="\"Nothing\", Default" w1006 {
              frame "Nothing", Default {
                n331 = local write "Y Length"(0) -> ()
                n332 = local write "X Length"(0) -> ()
                n333 = local write "Numeric"(2) -> ()
              }
              frame "Left" {
                n334 = local write "X Length"(0) -> ()
                n335 = local write "Y Length"(50) -> ()
              }
              frame "Top" {
                n336 = local write "X Length"(-50) -> ()
                n337 = local write "Y Length"(0) -> ()
              }
            }
            n338 = local write "Has encoders been reset?"(enum16{"don't reset", "reset"}."don't reset") -> ()
          }
          frame "reverse" {
            n339 = local write "Has encoders been reset?"(enum16{"don't reset", "reset"}."don't reset") -> ()
            "Numeric" <- 2
          }
        }
      }
    }
    "In drawing mode" <- w175
    n340 = case shown="True" w72 {
      tunnel: w152 -> [w482 w487]
      tunnel: w151 -> [w483 w486]
      tunnel: [w480 w485] -> w150
      frame False {
        n341 = call-poly <vilib>:"DAQmx Read.vi"("task/channels in"=w482, "error in"=w483) -> ("data"=w481:dbl, "error out"=w480:errorcluster)  [unwired: 11 in, 1 out]
        n342 = local write "Pulses M1"(w481) -> ()
      }
      frame True {
        n343 = case shown="\"don't reset\", Default" "Has encoders been reset?" {
          tunnel: w487 -> [w491 w498]
          tunnel: w486 -> [w490 w497]
          tunnel: [w488 w499] -> w485
          frame "don't reset", Default {
            n344 = call-poly <vilib>:"DAQmx Read.vi"("task/channels in"=w491, "error in"=w490) -> ("data"=→"Pulses M1":dbl, "error out"=w488:errorcluster)  [unwired: 11 in, 1 out]
          }
          frame "reset" {
            n345 = call <vilib>:"DAQmx Stop Task.vi"("task/channels in"=w498, "error in"=w497) -> ("task out"=w496:refnum<k21>, "error out"=w495:errorcluster)  [unwired: 12 in]
            n346 = call <vilib>:"DAQmx Start Task.vi"("task/channels in"=w496, "error in"=w495) -> ("task out"=w494:refnum<k21>, "error out"=w493:errorcluster)  [unwired: 12 in]
            n347 = call-poly <vilib>:"DAQmx Read.vi"("task/channels in"=w494, "error in"=w493) -> ("data"=w492:dbl, "error out"=w499:errorcluster)  [unwired: 11 in, 1 out]
            n348 = local write "Pulses M1"(w492) -> ()
          }
        }
      }
    }
    n349 = And(x=w96, y=w91) -> (x .and. y?=w158:bool)
    n350 = Or(x=w212, y=w158) -> (x .or. y?=w211:bool)
    n351 = Or(x=w211, y="Motor stop") -> (x .or. y?=w213:bool)
    n352 = Or(x=w213, y="stop") -> (x .or. y?=w233:bool)
    n353 = Select(t=0.0, s=w233, f=w84) -> (s? t:f=w230:dbl)
    n354 = call-poly <vilib>:"DAQmx Write.vi"("task/channels in"=w239, "data"=w230, "error in"=w236) -> ("task out"=w240:refnum<k21>, "error out"=w241:errorcluster)  [unwired: 10 in, 1 out]
    n355 = Select(t=0.0 ("s? t:f"), s=w233, f=w85) -> (s? t:f=w231:dbl)
    n356 = call-poly <vilib>:"DAQmx Write.vi"("task/channels in"=w245, "data"=w231, "error in"=w235) -> ("task out"=w244:refnum<k21>, "error out"=w243:errorcluster)  [unwired: 10 in, 1 out]
    n357 = call <vilib>:"DAQmx Wait Until Done.vi"("task/channels in"=w244, "error in"=w243) -> ("error out"=w242:errorcluster)  [unwired: 12 in, 1 out]
    n358 = call <vilib>:"DAQmx Wait Until Done.vi"("task/channels in"=w240, "error in"=w241) -> ("error out"=w238:errorcluster)  [unwired: 12 in, 1 out]
    n359 = case shown="True" w72 {
      tunnel: w148 -> [w471 w473]
      tunnel: w79 -> [_ w472]
      frame False {
        n360 = call-poly <vilib>:"DAQmx Read.vi"("task/channels in"=w471) -> ("data"=w470:dbl)  [unwired: 12 in, 2 out]
        n361 = local write "Pulses M2"(w470) -> ()
      }
      frame True {
        n362 = case shown="\"don't reset\", Default" w472 {
          tunnel: w473 -> [w475 w478]
          frame "don't reset", Default {
            n363 = call-poly <vilib>:"DAQmx Read.vi"("task/channels in"=w475) -> ("data"=→"Pulses M2":dbl)  [unwired: 12 in, 2 out]
          }
          frame "reset" {
            n364 = call <vilib>:"DAQmx Stop Task.vi"("task/channels in"=w478) -> ("task out"=w477:refnum<k21>)  [unwired: 13 in, 1 out]
            n365 = call <vilib>:"DAQmx Start Task.vi"("task/channels in"=w477) -> ("task out"=w479:refnum<k21>)  [unwired: 13 in, 1 out]
            n366 = call-poly <vilib>:"DAQmx Read.vi"("task/channels in"=w479) -> ("data"=w476:dbl)  [unwired: 12 in, 2 out]
            n367 = local write "Pulses M2"(w476) -> ()
          }
        }
      }
    }
    n368 = call "Number To Enum.vim"("number"=w171, "enum type"=enum16{"corner", "1st switch", "reverse"}."corner") -> ("number as enum"=→"Shape drawing steps":enum16{"corner", "1st switch", "reverse"})
  }
  n369 = invoke on="motor 1" class="Slide (strict)" method="Reinit To Default"() -> ()  [unwired: 3 in, 3 out]
  n370 = invoke on="Numeric" class="DigNum (strict)" method="Reinit To Default"() -> ()  [unwired: 3 in, 3 out]
  n371 = invoke on="No of Points" class="DigNum (strict)" method="Reinit To Default"() -> ()  [unwired: 3 in, 3 out]
  n372 = invoke on="Shape drawing steps" class="Enum (strict)" method="Reinit To Default"() -> ()  [unwired: 3 in, 3 out]
  n373 = invoke on="stage circle" class="Enum (strict)" method="Reinit To Default"() -> ()  [unwired: 3 in, 3 out]
  n374 = invoke on="array Y length 2" class="DigNum (strict)" method="Reinit To Default"() -> ()  [unwired: 3 in, 3 out]
  n375 = invoke on="array x Length 2" class="DigNum (strict)" method="Reinit To Default"() -> ()  [unwired: 3 in, 3 out]
  n376 = invoke on="Point circle is drawing" class="DigNum (strict)" method="Reinit To Default"() -> ()  [unwired: 3 in, 3 out]
  n377 = invoke on="previous index" class="DigNum (strict)" method="Reinit To Default"() -> ()  [unwired: 3 in, 3 out]
  n378 = call <vilib>:"Simple Error Handler.vi"("error source (\" \")"="you messed up" ("error source (\" \")"), "error in (no error)"=w48) -> ()  [unwired: 3 in, 5 out]
  n379 = call <vilib>:"Simple Error Handler.vi"("error source (\" \")"="you messed up" ("error source (\" \")"), "error in (no error)"=w45) -> ()  [unwired: 3 in, 5 out]
  n380 = call <vilib>:"DAQmx Clear Task.vi"("task in"=w27, "error in"=w25) -> ()  [unwired: 13 in, 1 out]
  n381 = call <vilib>:"DAQmx Clear Task.vi"("task in"=w17, "error in"=w14) -> ()  [unwired: 13 in, 1 out]
  n382 = call <vilib>:"DAQmx Clear Task.vi"("task in"=w18, "error in"=w15) -> ("error out"=w12:errorcluster)  [unwired: 13 in]
  n383 = call <vilib>:"DAQmx Clear Task.vi"("task in"=w16, "error in"=w13) -> ()  [unwired: 13 in, 1 out]
  n384 = call <vilib>:"Simple Error Handler.vi"("error in (no error)"=w12) -> ()  [unwired: 4 in, 5 out]
  n385 = call <vilib>:"Simple Error Handler.vi"("error source (\" \")"="you messed up" ("error source (\" \")"), "error in (no error)"=w10) -> ()  [unwired: 3 in, 5 out]
